vi "ImageTest.vi"() -> ()   [LabVIEW 2009]
uses:
  <vilib>/Robotics Library/NIFPGAInterface/DIO/PWMChannel.ctl
  <vilib>/addons/control/pid/pid.llb/PID Control Input Filter (DBL).vi
  <vilib>/Robotics Library/WPI/Camera/Camera.lvlib
  <vilib>/Robotics Library/WPI/PWM/Servo/Servo.lvlib
  <vilib>/addons/control/pid/NI_PID_pid.lvlib
  <vilib>/Robotics Library/WPI/PWM/PWM.lvlib
  <vilib>/Robotics Library/NIFPGAInterface/DIO/NIFPGA DIO.lvlib
panel:
  out "error out 3":errorcluster
  out "error out 2":errorcluster
  out "error out":errorcluster
  in  "stop 2":bool
  in  "stop":bool
  out "output":dbl
  in  "Loop Sleep 2":u32=20
  in  "Loop Sleep":u32=20
  in  "Servo Positions":cluster{"X":dbl, "Y":dbl}={"X"=85.52840986947938, "Y"=85.0} {"Y" scale=0.0..170.0; "X" scale=0.0..170.0}
  in  "Smooth":bool=TRUE
  in  "Y Channel":T1=enum."PWM 2"
  in  "X Channel":T1
  out "Image":T2(plugin-control)
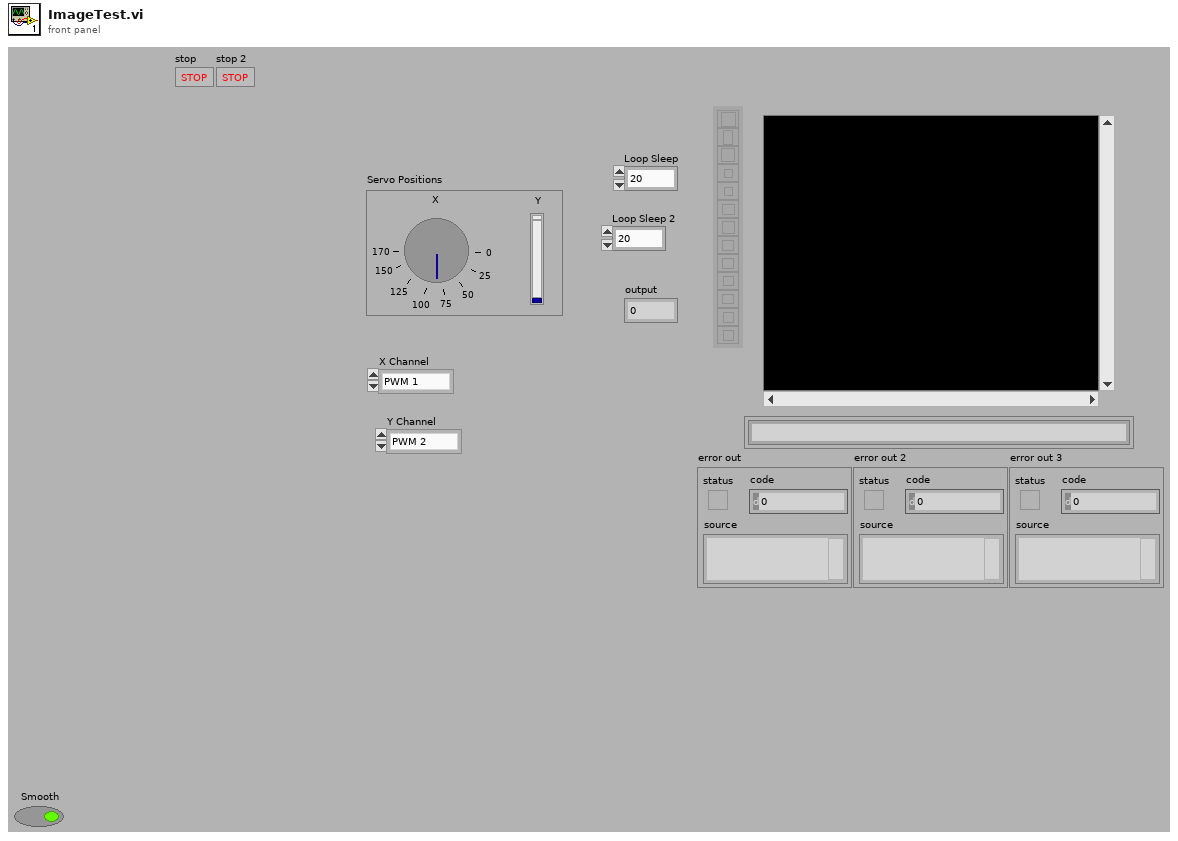
[diagram p1: front panel]
types:
  T1 = typedef "NI_FPGA_Interface.lvlib/NIFPGA DIO.lvlib/PWMChannel.ctl" = enum8{"PWM 1", "PWM 2", "PWM 3", "PWM 4", "PWM 5", "PWM 6", "PWM 7", "PWM 8", "PWM 9", "PWM 10", "Invalid"}
  T2 = typedef "IMAQ Image.ctl" = refnum<image>
  T3 = typedef "Image Type" = u32
  T4 = typedef "Camera.lvlib/CameraDevRef.ctl" = cluster{"Camera Address":string, "CameraStatus":errorcluster, "Session ID":T5}
  T5 = typedef "Camera.lvlib/SessionID.ctl" = i32
  T6 = typedef "PWM.lvlib/PWMDeviceRef.ctl" = cluster{"DeviceStatus":errorcluster, "DIO Module":T7, "PWM Channel":T1, "Invert":bool, "TransformRef":T8, "InvTransformRef":T8, "DeadBand":T9}
  T7 = typedef "NI_FPGA_Interface.lvlib/DigitalModule.ctl" = enum16{"Default", "Slot 4", "Slot 6"}
  T8 = typedef "PWM.lvlib/Transform_ConPane.ctl" = refnum<vi>
  T9 = typedef "PWM.lvlib/Deadband.ctl" = cluster{"Name":string, "maxPositivePwm":i32, "minPositivePwm":i32, "centerPwm":i32, "maxNegativePwm":i32, "minNegativePwm":i32, "angularRange":u16}
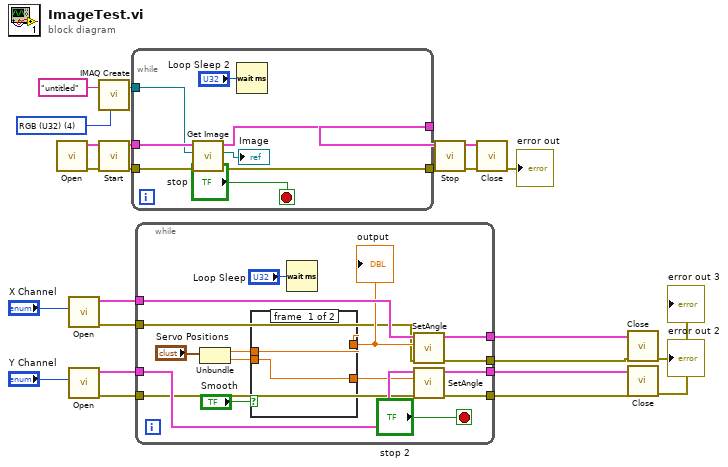
[diagram p0: block diagram]
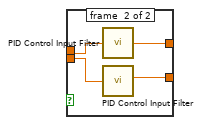
[diagram p2: hidden frame]
diagram:
  w18 = T3 4 items=["Grayscale (U8)", "Grayscale (I16)", "Grayscale (SGL)", "Complex (CSG)", "RGB (U32)", "HSL (U32)", "RGB (U64)", "Grayscale (U16)"] ("Image Type")
  n1 = call <vilib>:"Open.vi"() -> ("error out"=w23:errorcluster, "CameraDevRef"=w24:T4)  [unwired: 10 in]
  n2 = call <vilib>:"Open.vi"("PWM Channel"="X Channel") -> ("error out"=w6:errorcluster, "PWMDeviceRef"=w11:T6)  [unwired: 9 in]
  n3 = call <vilib>:"Open.vi"("PWM Channel"="Y Channel") -> ("error out"=w3:errorcluster, "PWMDeviceRef"=w9:T6)  [unwired: 9 in]
  n4 = call "IMAQ Create"("Image Name"="untitled", "Image Type"=w18) -> ("New Image"=w20:T2)  [unwired: 3 in, 1 out]
  n5 = call <vilib>:"Start.vi"("error in (no error)"=w23, "CameraDevRef"=w24) -> ("error out"=w21:errorcluster, "CameraDevRef Out"=w22:T4)  [unwired: 8 in]
  n6 = while {
    tunnel: w22 -> [w32]
    tunnel: w21 -> [w31]
    tunnel: [w29] -> w17
    tunnel: [w28] -> w16
    tunnel: w20 -> [w30]
    stop <- "stop" stop-if-true
    n7 = call <vilib>:"Get Image.vi"("error in (no error)"=w31, "Image"=w30, "CameraDevRef"=w32) -> ("error out"=w28:errorcluster, "Image Out"=→"Image":T2, "CameraDevRef Out"=w29:T4)  [unwired: 6 in]
    n8 = Wait (ms)(milliseconds to wait="Loop Sleep 2") -> ()  [unwired: 1 out]
  }
  n9 = while {
    tunnel: w11 -> [w46]
    tunnel: [w48] -> w10
    tunnel: w9 -> [w45]
    tunnel: [w44] -> w8
    tunnel: w6 -> [w36]
    tunnel: [w35] -> w5
    tunnel: w3 -> [w34]
    tunnel: [w33] -> w2
    stop <- "stop 2" stop-if-true
    n10 = Unbundle("Servo Positions") -> ("X"=w42:dbl, "Y"=w40:dbl)
    n11 = case shown="True" "Smooth" {
      tunnel: w42 -> [w50 w54]
      tunnel: [w50 w53] -> w41
      tunnel: w40 -> [w49 w52]
      tunnel: [w49 w51] -> w39
      frame #0 {
      }
      frame #1 {
        n12 = call-poly <vilib>:"PID Control Input Filter.vi"("input"=w54) -> ("output"=w53:dbl)  [unwired: 4 in]
        n13 = call-poly <vilib>:"PID Control Input Filter.vi"("input"=w52) -> ("output"=w51:dbl)  [unwired: 4 in]
      }
    }
    "output" <- w41
    n14 = Wait (ms)(milliseconds to wait="Loop Sleep") -> ()  [unwired: 1 out]
    n15 = call <vilib>:"SetAngle.vi"("error in (no error)"=w36, "Angle"=w41, "PWMDeviceRef"=w46) -> ("error out"=w35:errorcluster, "PWMDeviceRef"=w48:T6)  [unwired: 7 in]
    n16 = call <vilib>:"SetAngle.vi"("error in (no error)"=w34, "Angle"=w39, "PWMDeviceRef"=w45) -> ("error out"=w33:errorcluster, "PWMDeviceRef"=w44:T6)  [unwired: 7 in]
  }
  n17 = call <vilib>:"Stop.vi"("error in (no error)"=w16, "CameraDevRef"=w17) -> ("error out"=w15:errorcluster, "CameraDevRef Out"=w14:T4)  [unwired: 8 in]
  n18 = call <vilib>:"Close.vi"("error in (no error)"=w15, "CameraDevRef"=w14) -> ("error out"=→"error out":errorcluster)  [unwired: 9 in]
  n19 = call <vilib>:"Close.vi"("error in (no error)"=w5, "PWMDeviceRef"=w10) -> ("error out"=→"error out 2":errorcluster)  [unwired: 9 in]
  n20 = call <vilib>:"Close.vi"("error in (no error)"=w2, "PWMDeviceRef"=w8) -> ("error out"=→"error out 3":errorcluster)  [unwired: 9 in]
